vi "Calibrate_AOL XYZ.vi"(5 "Symmetric":bool, 7 "FOV/Z Range":i32=5, 8 "error in (no error)":errorcluster, 10 "number of points":i32=5, 11 "Stage Control":T1=enum."XY-Y") -> (0 "error out":errorcluster, 2 "norm_to_um_scaling":dbl)   [LabVIEW 2020]
doc: "Use this template to create a dialog box with event handling."
uses:
  TypeDefs/Control Plane.ctl
  Typedefs/Top level VI states.ctl
  Peripherals Control/XYZ Stage/Typedefs/XYZ stage states.ctl
  Peripherals Control/XYZ Stage/Typedefs/XYZ stage data.ctl
  Peripherals Control/XYZ Stage/Typedefs/XYZ channel ring.ctl
  Globals/gl_Calibration globals.vi
  Global Variables/General Globals.vi
panel:
  in  "Delay":u32=1000
  out "Cal":sgl[][](array[numeric])
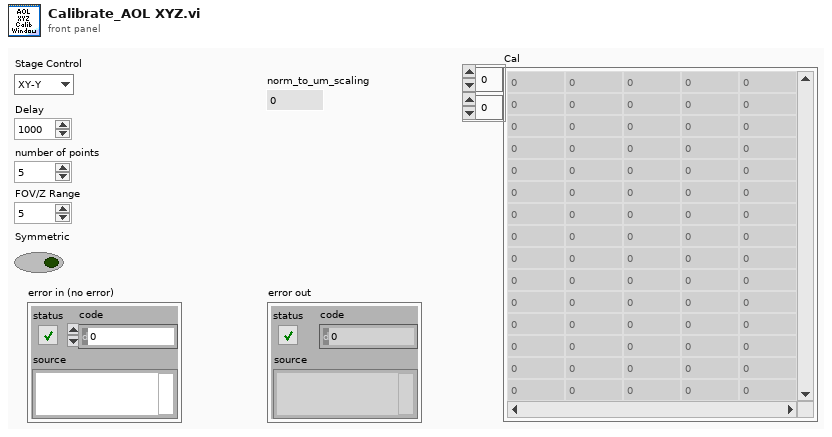
[diagram p1: front panel]
types:
  T1 = typedef "Control Plane.ctl" = enum16{"XY-X", "XY-Y", "Z"}
  T2 = typedef "Top level VI states.ctl" = enum16{"None", "Initialise UI", "<STACK PROTOCOL STATES>", "AOL Zstack-START", "AOL Zstack-STOP", "Motor Zstack-START", "Motor Zstack-STOP", "<ACQUISITION PROTOCOL STATES> ", "Functional Acquisition-START", "Functional Acquisition-STOP", "Single Plane Acquisition-START", "Single Plane Acquisition-STOP", "Volume Acquisition-START", "Volume Acquisition-STOP", "<LIVE IMAGING PROTOCOL STATES>", "Live Imaging-START", "Live Imaging-STOP", "Live Plane Imaging-START", "Live Plane Imaging-STOP", "Live Volume Imaging-START", "Live Volume Imaging-STOP", "<MOVEMENT CORRECTION PROTOCOL STATES>", "EXIT"}
  T3 = typedef "XYZ channel ring.ctl" = string
  T4 = typedef "XYZ stage data.ctl" = cluster{"Command":T5, "Channel":T3, "X":sgl, "Y":sgl, "Z":sgl, "Speed":i32, "Zero":bool, "Use acknowledgement?":bool}
  T5 = typedef "XYZ stage states.ctl" = enum16{"Dequeue", "Initialize", "Read Position", "Read Speed Setting", "Move", "Set Max Speed", "Reset Axis", "Stop all movement"}
  T6 = typedef "General Scan Parameters.ctl" = cluster{"Field of View":sgl, "Frame Size":u16, "Dwell Time (ms)":dbl, "Wavelength (nm)":dbl, "Zoom":dbl, "AOL Xc":sgl, "AOL Yc":sgl, "AOL Zc":sgl, "AOL Mode":enum16{"Raster", "Structural", "Pointing", "Mini Scan", "Alignment"}, "Imaging Mode":enum16{"Live Imaging", "AOL Zstack", "Motor Zstack", "Functional Imaging"}}
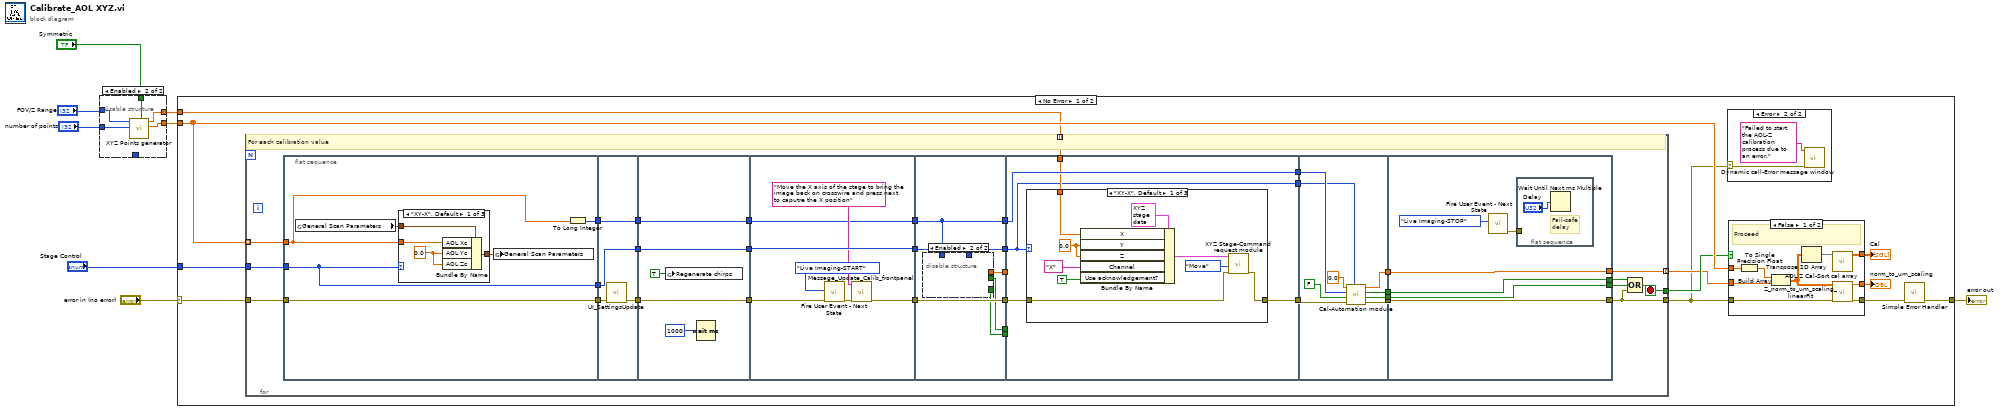
[diagram p0: block diagram]
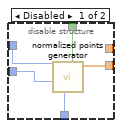
[diagram p2: hidden frame]
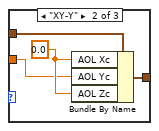
[diagram p3: hidden frame]
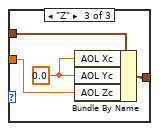
[diagram p4: hidden frame]
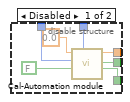
[diagram p5: hidden frame]
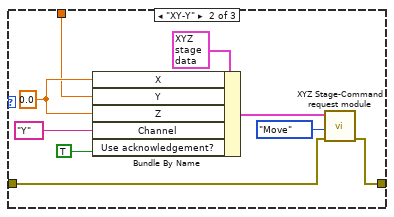
[diagram p6: hidden frame]
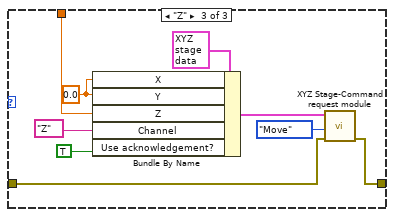
[diagram p7: hidden frame]
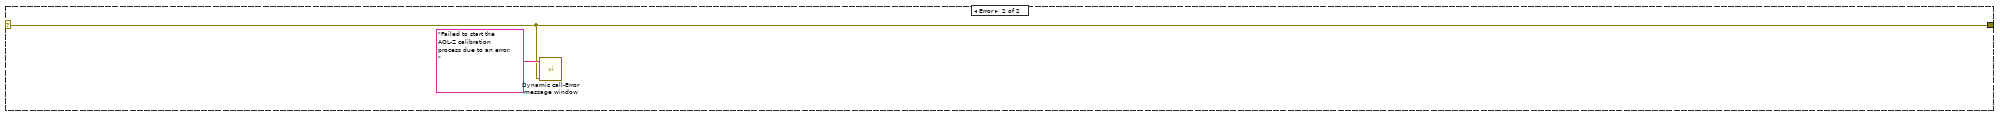
[diagram p10: hidden frame]
diagram:
  n1 = disable-structure shown="Enabled" {
    disable-tunnel: [w13 w15] -> w6
    disable-tunnel: "number of points" -> [w12 w16]
    disable-tunnel: "Symmetric" -> [w11 w18]
    disable-tunnel: _ -> [w10 _]
    disable-tunnel: "FOV/Z Range" -> [w9 w17]
    disable-tunnel: [_ w14] -> w1
    frame Disabled {
      n2 = call "normalized points generator.vi"("Symmetric"=w11, "Stage Control"=w10, "FOV(real)"=w9, "number of points"=w12) -> ("normalised array"=w13:dbl[])  [unwired: 6 in, 1 out]
    }
    frame Enabled {
      n3 = call "XYZ Points generator.vi"("Symmetric"=w18, "Number of points"=w16, "FOV/ Z-range"=w17) -> ("Normalised centre Points"=w15:dbl[], "Stage Points"=w14:dbl[])  [unwired: 7 in]
    }
  }
  n4 = case shown="No Error" "error in (no error)" {
    selector: "error in (no error)" -> [w21 w171]
    tunnel: w6 -> [w29 _]
    tunnel: [w26 w171] -> w8
    tunnel: "Stage Control" -> [w23 _]
    tunnel: w1 -> [w19 _]
    frame No Error {
      n5 = for {
        tunnel: w29 -> [w62] mode=indexing
        tunnel: [w63] -> w25 mode=indexing
        tunnel: [w54] -> w27
        tunnel: [w55] -> w24
        tunnel: w21 -> [w60]
        tunnel: w23 -> [w58]
        tunnel: w19 -> [w39] mode=indexing
        stop <- w54 stop-if-true
        # "For each calibration value"
        n6 = flat-sequence {
          tunnel: w62 -> [w65]
          tunnel: w60 -> [w66]
          tunnel: [w66] -> w59
          tunnel: w58 -> [w67]
          tunnel: [w67] -> w56
          tunnel: [w64] -> w48
          tunnel: w59 -> [w85]
          tunnel: [w84] -> w45
          tunnel: w56 -> [w84]
          tunnel: [w82] -> w43
          tunnel: w48 -> [w83]
          tunnel: [w83] -> w41
          tunnel: w45 -> [w90]
          tunnel: [w90] -> w44
          tunnel: w43 -> [w89]
          tunnel: [w89] -> w42
          tunnel: w41 -> [w88]
          tunnel: [w88] -> w40
          tunnel: [w95] -> w61
          tunnel: [w96] -> w57
          tunnel: w44 -> [w96]
          tunnel: w42 -> [w97]
          tunnel: w40 -> [w92]
          tunnel: [w92] -> w47
          tunnel: [w102] -> w53
          tunnel: [w103] -> w52
          tunnel: w61 -> [w103]
          tunnel: w57 -> [w98]
          tunnel: [w100] -> w51
          tunnel: [w101] -> w50
          tunnel: [w98] -> w49
          tunnel: w47 -> [w99]
          tunnel: [w99] -> w46
          tunnel: w53 -> [_]
          tunnel: w52 -> [w115]
          tunnel: [w114] -> w37
          tunnel: w51 -> [_]
          tunnel: w50 -> [_]
          tunnel: w49 -> [w111]
          tunnel: w46 -> [w113]
          tunnel: [w113] -> w35
          tunnel: w39 -> [w112]
          tunnel: [w111] -> w34
          tunnel: [w145] -> w38
          tunnel: w37 -> [w149]
          tunnel: [w148] -> w36
          tunnel: w35 -> [w147]
          tunnel: w34 -> [w146]
          tunnel: [w144] -> w32
          tunnel: [w143] -> w31
          tunnel: [w156] -> w63
          tunnel: w38 -> [w156]
          tunnel: w36 -> [w155]
          tunnel: [w155] -> w55
          tunnel: [w153] -> w33
          tunnel: w32 -> [w153]
          tunnel: w31 -> [w152]
          tunnel: [w152] -> w30
          frame #0 {
            n7 = global read "gl_Calibration globals.vi" "General Scan Parameters"() -> (w69:T6)
            n8 = case shown="\"XY-X\", Default" w67 {
              tunnel: w69 -> [w70 w77 w81]
              tunnel: [w73 w76 w80] -> w68
              tunnel: w65 -> [w72 w74 w78]
              frame "XY-X", Default {
                w71 = sgl 0.0 ("AOL Yc")
                n9 = Bundle By Name(cluster=w70, "AOL Xc"=w72, "AOL Yc"=w71, "AOL Zc"=w71) -> (w73:T6)
              }
              frame "XY-Y" {
                w75 = sgl 0.0 ("AOL Xc")
                n10 = Bundle By Name(cluster=w77, "AOL Xc"=w75, "AOL Yc"=w74, "AOL Zc"=w75) -> (w76:T6)
              }
              frame "Z" {
                w79 = sgl 0.0 ("AOL Xc")
                n11 = Bundle By Name(cluster=w81, "AOL Xc"=w79, "AOL Yc"=w79, "AOL Zc"=w78) -> (w80:T6)
              }
            }
            n12 = global write "gl_Calibration globals.vi" "General Scan Parameters"(w68) -> ()
            n13 = To Long Integer(number=w65) -> (32bit integer=w64:i32)
          }
          frame #1 {
            n14 = call "UI_SettingsUpdate.vi"("error in (no error)"=w85) -> ("error out"=w82:errorcluster)  [unwired: 10 in]
          }
          frame #2 {
            n15 = global write "General Globals.vi" "Regenerate chirps"(TRUE ("Regenerate chirps")) -> ()
            n16 = Wait (ms)(milliseconds to wait=u32 1000) -> ()  [unwired: 1 out]
          }
          frame #3 {
            n17 = call "Fire User Event - Next State.vi"("Error In"=w97, "\"UI Handler loop\" case to execute"=Top_level_VI_states."Live Imaging-START" ("\"UI Handler loop\" case to execute")) -> ("Error Out"=w94:errorcluster)  [unwired: 9 in]
            n18 = call "Message_Update_Calib_frontpanel.vi"("error in (no error)"=w94, "Message"="Move the X axis of the stage to bring the image back on crosswire and press next to caputre the X position") -> ("error out"=w95:errorcluster)  [unwired: 9 in]
          }
          frame #4 {
            n19 = disable-structure shown="Enabled" {
              disable-tunnel: [w110 _] -> w102
              disable-tunnel: [w107 _] -> w101
              disable-tunnel: [w106 _] -> w100
              disable-tunnel: w99 -> [w105 _]
              disable-tunnel: w98 -> [w104 _]
              frame Disabled {
                n20 = call "Cal-Automation module.vi"("Parameter"=w104, "Timed out while waiting for acknowledgement in"=FALSE, "FOR loop index"=w105, "Initial motor position (um)"=sgl 0.0) -> ("Motor timed out or errored out"=w106:bool, "Cancelled"=w107:bool, "Measured cal value"=w110:sgl)  [unwired: 4 in, 1 out]
              }
              frame Enabled {
              }
            }
          }
          frame #5 {
            n21 = case shown="\"XY-X\", Default" w111 {
              tunnel: w115 -> [w119 w129 w138]
              tunnel: [w118 w128 w137] -> w114
              tunnel: w112 -> [w117 w126 w135]
              frame "XY-X", Default {
                w123 = 0.0
                n22 = Bundle By Name(cluster=T4 {"Command"=enum."Initialize", "Channel"="", "X"=0.0, "Y"=0.0, "Z"=0.0, "Speed"=0, "Zero"=TRUE, "Use acknowledgement?"=FALSE} ("XYZ Stage data to queue"), "X"=w117, "Y"=w123, "Z"=w123, "Channel"=T3 "X", "Use acknowledgement?"=TRUE ("Wait for acknowledge?")) -> (w124:T4)
                n23 = call "XYZ Stage-Command request module.vi"("error in"=w119, "Command"=XYZ_stage_states."Move", "XYZ Stage data to queue"=w124) -> ("error out"=w118:errorcluster)  [unwired: 4 in, 4 out]
              }
              frame "XY-Y" {
                w127 = 0.0
                n24 = Bundle By Name(cluster=T4 {"Command"=enum."Initialize", "Channel"="", "X"=0.0, "Y"=0.0, "Z"=0.0, "Speed"=0, "Zero"=TRUE, "Use acknowledgement?"=FALSE} ("XYZ Stage data to queue"), "X"=w127, "Y"=w126, "Z"=w127, "Channel"=T3 "Y", "Use acknowledgement?"=TRUE ("Wait for acknowledge?")) -> (w133:T4)
                n25 = call "XYZ Stage-Command request module.vi"("error in"=w129, "Command"=XYZ_stage_states."Move", "XYZ Stage data to queue"=w133) -> ("error out"=w128:errorcluster)  [unwired: 4 in, 4 out]
              }
              frame "Z" {
                w136 = 0.0
                n26 = Bundle By Name(cluster=T4 {"Command"=enum."Initialize", "Channel"="", "X"=0.0, "Y"=0.0, "Z"=0.0, "Speed"=0, "Zero"=TRUE, "Use acknowledgement?"=FALSE} ("XYZ Stage data to queue"), "X"=w136, "Y"=w136, "Z"=w135, "Channel"=T3 "Z", "Use acknowledgement?"=TRUE ("Wait for acknowledge?")) -> (w142:T4)
                n27 = call "XYZ Stage-Command request module.vi"("error in"=w138, "Command"=XYZ_stage_states."Move", "XYZ Stage data to queue"=w142) -> ("error out"=w137:errorcluster)  [unwired: 4 in, 4 out]
              }
            }
          }
          frame #6 {
            n28 = call "Cal-Automation module.vi"("Parameter"=w146, "error in (no error)"=w149, "Timed out while waiting for acknowledgement in"=FALSE, "FOR loop index"=w147, "Initial motor position (um)"=sgl 0.0) -> ("error out"=w148:errorcluster, "Motor timed out or errored out"=w143:bool, "Cancelled"=w144:bool, "Measured cal value"=w145:sgl)  [unwired: 3 in]
          }
          frame #7 {
            n29 = call "Fire User Event - Next State.vi"("\"UI Handler loop\" case to execute"=Top_level_VI_states."Live Imaging-STOP" ("\"UI Handler loop\" case to execute")) -> ("Error Out"=w157:errorcluster)  [unwired: 10 in]
            n30 = flat-sequence {
              tunnel: w157 -> [_]
              frame #0 {
                # "Fail-safe delay"
                n31 = Wait Until Next ms Multiple(millisecond multiple="Delay") -> ()  [unwired: 1 out]
              }
            }
          }
        }
        n32 = Compound Arithmetic op=OR(w33, w30, w55) -> (w54:bool)
      }
      n33 = case shown="Error" w24 {
        selector: w24 -> [_ w160]
        frame No Error {
        }
        frame Error {
          n34 = call "Dynamic call-Error message window.vi"("error in (no error)"=w160, "Error Message"="Failed to start the AOL-Z calibration process due to an error.") -> ()  [unwired: 9 in, 1 out]
        }
      }
      n35 = case shown="False" w27 {
        tunnel: w29 -> [w169 _]
        tunnel: w25 -> [w168 _]
        tunnel: [w167 _] -> w20
        tunnel: [w165 w170] -> w28
        tunnel: w24 -> [w164 w170]
        tunnel: [w163 _] -> w22
        frame False {
          # "Proceed"
          n36 = To Single Precision Float(number=w169) -> (single precision float=w166:sgl[])
          n37 = Build Array(w166, w168) -> (w161:sgl[][])
          n38 = Transpose 2D Array(2D array=w161) -> (transposed array=w162:sgl[][])
          n39 = call "AOL Z Cal-Sort cal array.vi"("Unsorted cal"=w162) -> ("Sorted cal"=w167:sgl[][])  [unwired: 10 in]
          n40 = call "Z_norm_to_um_scaling_linearFit.vi"("Input Array(Znorm, Z_um)"=w161, "error in (no error)"=w164) -> ("Znorm_to_um_scaling"=w163:dbl, "error out"=w165:errorcluster)  [unwired: 7 in]
        }
        frame True {
          # "Cancelled/Aborted"
        }
      }
      "Cal" <- w20
      "norm_to_um_scaling" <- w22
      n41 = call <vilib>:"Simple Error Handler.vi"("error in (no error)"=w28) -> ("error out"=w26:errorcluster)  [unwired: 4 in, 4 out]
    }
    frame Error {
      n42 = call "Dynamic call-Error message window.vi"("error in (no error)"=w171, "Error Message"="Failed to start the AOL-Z calibration process due to an error.") -> ()  [unwired: 9 in, 1 out]
    }
  }
  "error out" <- w8
